vi "rystr_join_integers.vi"(0 "elements":i32[](array[numeric]), 1 "delimiter (',')":string=",") -> (6 "string":string)   [LabVIEW 2017]
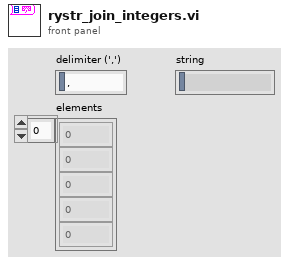
[diagram p1: front panel]
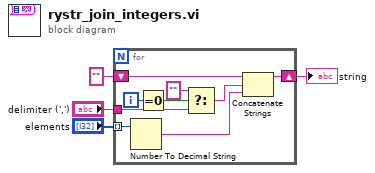
[diagram p0: block diagram]
diagram:
  n1 = for {
    tunnel: "elements" -> [w13] mode=indexing
    shift-right: [w11] -> w1
    shift-left: "" -> [w12]
    tunnel: "delimiter (',')" -> [w7]
    i -> [w10]
    n2 = Number To Decimal String(number=w13) -> (decimal integer string=w5:string)  [unwired: 1 in]
    n3 = Equal To 0?(x=w10) -> (x = 0?=w9:bool)
    n4 = Select(t="", s=w9, f=w7) -> (s? t:f=w6:string)
    n5 = Concatenate Strings(w12, w6, w5) -> (w11:string)
  }
  "string" <- w1
